vi "多参数传感器参数读取.vi"(8 "Error in":errorcluster caption="Error in (no error)") -> (0 "error out":errorcluster, 3 "添加的数组":string[][](array[string]))   [LabVIEW 2016, in "斯坦道仪器.lvlib"]
panel:
  in  "传感器区":i32(listbox)
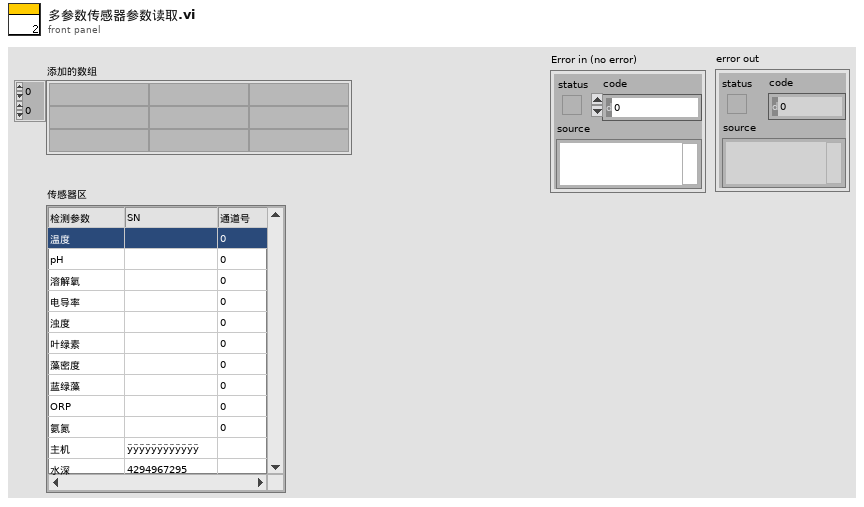
[diagram p1: front panel]
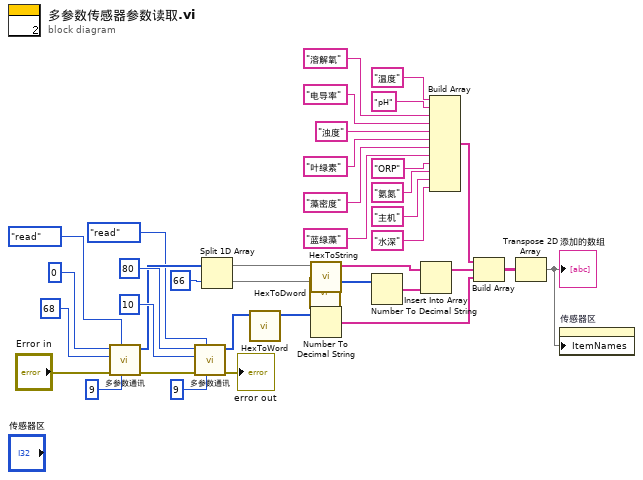
[diagram p0: block diagram]
diagram:
  n1 = call "多参数通讯.vi"("Slave ID"=u8 9, "STEP"=enum16{"open", "read", "write", "close"}."read", "Error in"="Error in", "quantity"=u16 68, "starting address"=u16 0) -> ("error out"=w35:errorcluster, "Registers"=w32:u16[])  [unwired: 4 in, 1 out]
  n2 = call "多参数通讯.vi"("Slave ID"=u8 9, "STEP"=enum16{"open", "read", "write", "close"}."read", "Error in"=w35, "quantity"=u16 10, "starting address"=u16 80) -> ("error out"=→"error out":errorcluster, "Registers"=w8:u16[])  [unwired: 4 in, 1 out]
  n3 = Split 1D Array(array=w32, index=66 ("索引")) -> (first subarray=w30:u16[], second subarray=w6:u16[])
  n4 = call "HexToWord.vi"("数组"=w8) -> ("WORD"=w7:u16[])  [unwired: 10 in]
  n5 = call "HexToDword.vi"("数组"=w6) -> ("DWORD"=w5:i32[])  [unwired: 10 in]
  n6 = call "HexToString.vi"("数组"=w30) -> ("STRING"=w17:string[])  [unwired: 10 in]
  n7 = Number To Decimal String(number=w7) -> (decimal integer string=w13:string[])  [unwired: 1 in]
  n8 = Number To Decimal String(number=w5) -> (decimal integer string=w16:string[])  [unwired: 1 in]
  n9 = Insert Into Array(array=w17, new element=w16) -> (w14:string[])  [unwired: 1 in]
  n10 = Build Array("温度", "pH", "溶解氧", "电导率", "浊度", "叶绿素", "藻密度", "蓝绿藻", "ORP", "氨氮", "主机", "水深") -> (w15:string[])
  n11 = Build Array(w15, w14, w13) -> (w12:string[][])
  n12 = Transpose 2D Array(2D array=w12) -> (transposed array=w11:string[][])
  "添加的数组" <- w11
  n13 = property on="传感器区" class="MCListbox (严格)"("ItemNames"=w11) -> ()  [unwired: 2 in, 2 out]
